vi "Skip DQMH Uis.vi"(8 "Action":enum16{"Read", "Write", "Delete"}(ring), 11 "Skip DQMH UIs":bool) -> (3 "Skip DQMH UIs":bool)   [LabVIEW 2020, in "Panther Dashboard.lvlib"]
doc: "The intention of this VI is to\nEnable/Disable Panther Dashboard\nUIS, when Disabled, the Default\nDQMH UIs will be Used"
uses:
  Panther Dashboard.lvlib
  <resource>/dialog/lvconfig.llb/LV Config Read Boolean.vi
  <resource>/dialog/lvconfig.llb/LV Config Write Boolean.vi
panel:
  out "error out":errorcluster
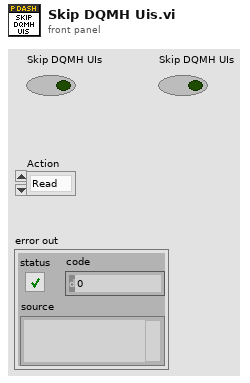
[diagram p1: front panel]
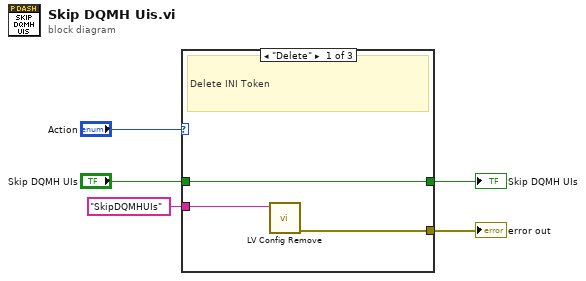
[diagram p0: block diagram]
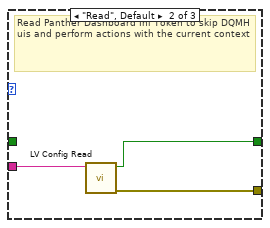
[diagram p2: hidden frame]
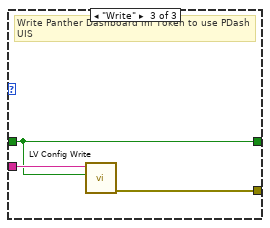
[diagram p3: hidden frame]
diagram:
  n1 = case shown="\"Delete\"" "Action" {
    tunnel: "SkipDQMHUIs" ("key") -> [w6 w10 w13]
    tunnel: "Skip DQMH UIs" -> [w7 _ w12]
    tunnel: [w7 w9 w12] -> w2
    tunnel: [w8 w11 w14] -> w5
    frame "Delete" {
      # "Delete INI Token"
      n2 = call <resource>:"LV Config Remove.vi"("key"=w6) -> ("error out"=w8:errorcluster)  [unwired: 6 in]
    }
    frame "Read", Default {
      # "Read Panther Dashboard Ini Token to skip DQMH uis and perform actions with the current context"
      n3 = call-poly <resource>:"LV Config Read.vi"("key"=w10) -> ("error out"=w11:errorcluster, "value"=w9:bool)  [unwired: 4 in, 1 out]
    }
    frame "Write" {
      # "Write Panther Dashboard Ini Token to use PDash UIS"
      n4 = call-poly <resource>:"LV Config Write.vi"("value"=w12, "key"=w13) -> ("error out"=w14:errorcluster)  [unwired: 5 in]
    }
  }
  "Skip DQMH UIs" <- w2
  "error out" <- w5
